vi "oa_Check dr Greater Than Zero.vi"(8 "error in (no error)":errorcluster, 11 "resampled signal":cluster{"r0":dbl, "dr":dbl, "Y":dbl[]} {"r0" format="%.2p"; "dr" format="%.2p"; "Y" format="%.2f"}) -> (0 "error out":errorcluster, 3 "resampled signal dup":cluster{"r0":dbl, "dr":dbl, "Y":dbl[]} {"r0" format="%.2p"; "dr" format="%.2p"; "Y" format="%.2f"})   [LabVIEW 2017, in "SoundVib_Resampling.lvlib"]
uses:
  <vilib>/addons/Sound and Vibration/Order Analysis/Resample Order Tracking/SoundVib_Resampling.lvlib
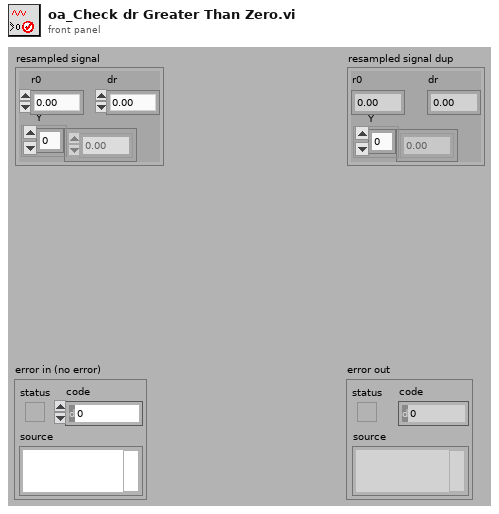
[diagram p1: front panel]
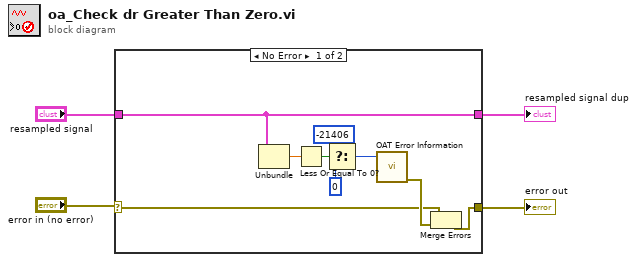
[diagram p0: block diagram]
diagram:
  n1 = case shown="No Error" "error in (no error)" {
    selector: "error in (no error)" -> [w5 w15]
    tunnel: [w7 w15] -> w3
    tunnel: "resampled signal" -> [w8 w14]
    tunnel: [w8 w14] -> w1
    frame No Error {
      n2 = Unbundle(w8) -> ("dr"=w13:dbl)  [unwired: 2 out]
      n3 = Less Or Equal To 0?(x=w13) -> (x <= 0?=w12:bool)
      n4 = Select(t=-21406, s=w12, f=0) -> (s? t:f=w10:i32)
      n5 = call <vilib>:"OAT Error Information.vi"("error code"=w10) -> ("error out"=w6:errorcluster)  [unwired: 6 in]
      n6 = Merge Errors(w5, w6) -> (w7:errorcluster)
    }
    frame Error {
    }
  }
  "error out" <- w3
  "resampled signal dup" <- w1
